vi "MICSD Start Session.vi"(8 "error in (no error)":errorcluster, 9 "Enable Watchdog?(T)":bool=TRUE, 10 "Wait Time (S)":u8=4, 11 "VISA Resource Name":refnum<visa-resource-name>) -> (0 "error out":errorcluster, 3 "dup VISA Resource Name":refnum<visa-resource-name>)   [LabVIEW 2020]
uses:
  <vilib>/Instr/_visa.llb/VISA Configure Serial Port (Instr).vi
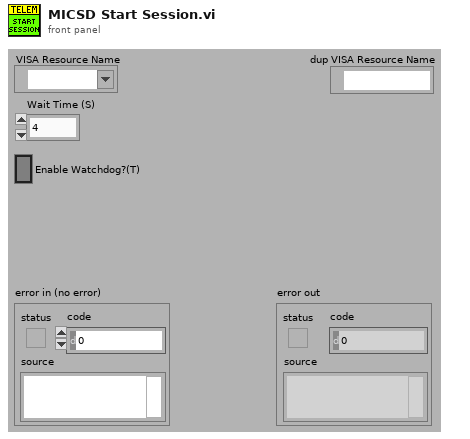
[diagram p1: front panel]
types:
  T1 = cluster{"Command Token":u8, "Length":u16, "Pack Data":u8[]}
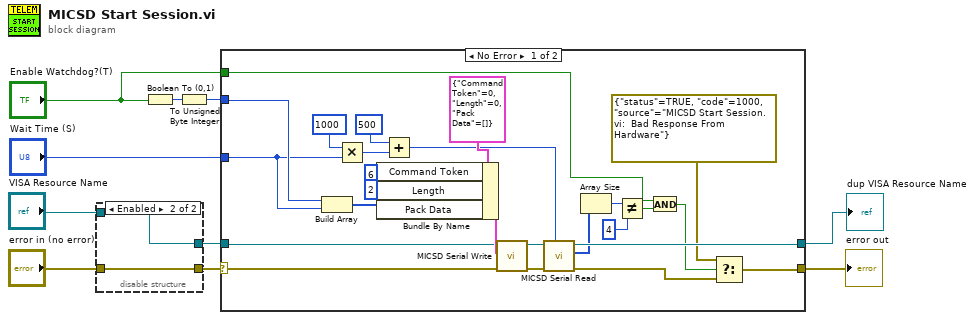
[diagram p0: block diagram]
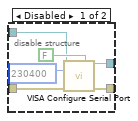
[diagram p2: hidden frame]
diagram:
  n1 = disable-structure shown="Enabled" {
    disable-tunnel: [w14 w17] -> w6
    disable-tunnel: "error in (no error)" -> [w13 w17]
    disable-tunnel: "VISA Resource Name" -> [w12 w18]
    disable-tunnel: [w11 w18] -> w3
    frame Disabled {
      n2 = call-poly "VISA Configure Serial Port"("VISA resource name"=w12, "Enable Termination\nChar (T)"=FALSE ("Enable Termination\nChar (T)"), "baud rate (9600)"=u32 230400, "error in (no error)"=w13) -> ("VISA resource name out"=w11:refnum<visa-resource-name>, "error out"=w14:errorcluster)  [unwired: 10 in]
    }
    frame Enabled {
    }
  }
  n3 = Boolean To (0,1)(Boolean="Enable Watchdog?(T)") -> (0, 1=w9:i16)
  n4 = To Unsigned Byte Integer(number=w9) -> (unsigned 8bit integer=w8:u8)
  n5 = case shown="No Error" w6 {
    selector: w6 -> [w38 w45]
    tunnel: [w43 w45] -> w2
    tunnel: w3 -> [w37 w44]
    tunnel: [w34 w44] -> w7
    tunnel: "Wait Time (S)" -> [w31 _]
    tunnel: w8 -> [w35 _]
    tunnel: "Enable Watchdog?(T)" -> [w20 _]
    frame No Error {
      n6 = Build Array(w35, w31) -> (w36:u8[])
      n7 = Multiply(x=u16 1000, y=w31) -> (x*y=w29:u16)
      n8 = Bundle By Name(cluster=T1 {"Command Token"=0, "Length"=0, "Pack Data"=[]} ("Write Data"), "Command Token"=u8 6, "Length"=u16 2, "Pack Data"=w36) -> (w42:T1)
      n9 = Add(x=u16 500, y=w29) -> (x+y=w22:u16)
      n10 = call "MICSD Serial Write.vi"("error in (no error)"=w38, "Write Data"=w42, "VISA Resource Name"=w37) -> ("error out"=w33:errorcluster, "DUP Visa Resource Name"=w32:refnum<visa-resource-name>)  [unwired: 7 in]
      n11 = call "MICSD Serial Read.vi"("Timeout(mS)"=w22, "error in (no error)"=w33, "VISA Resource Name"=w32) -> ("error out"=w26:errorcluster, "Read Data"=w25:u8[], "DUP Visa Resource Name"=w34:refnum<visa-resource-name>)  [unwired: 6 in]
      n12 = Array Size(array=w25) -> (size(s)=w24:i32)
      n13 = Not Equal?(x=w24, y=4) -> (x != y?=w21:bool)
      n14 = And(x=w20, y=w21) -> (x .and. y?=w19:bool)
      n15 = Select(t=errorcluster {"status"=TRUE, "code"=1000, "source"="MICSD Start Session.vi:  Bad Response From Hardware"} ("error IO"), s=w19, f=w26) -> (s? t:f=w43:errorcluster)
    }
    frame Error {
    }
  }
  "dup VISA Resource Name" <- w7
  "error out" <- w2
